vi "Configure Output Voltage.vi"(0 "VISA resource name":refnum<visa-resource-name>, 2 "Communication Address (0)":i16 max=254 format="%x", 7 "Output Voltage (0)":dbl min=0.0 max=18.0 format="%#.2g", 11 "error in (no error)":errorcluster) -> (4 "VISA resource name out":refnum<visa-resource-name>, 15 "error out":errorcluster)   [LabVIEW 2015, in "BK Precision 178XB Series.lvlib"]
doc: "This VI configures the output voltage. The valid range depends on the maximum output voltage set using <b>Configure Max Output Voltage.vi</b>."
uses:
  <instrlib>/BK Precision 178XB Series/BK Precision 178XB Series.lvlib
panel:
  # "(c) 2009 B&K PRECISION CORPORATION.  ALL RIGHTS RESERVED."
  # "Note:  The allowable Output Voltage to be set is based on the maximum output voltage configured using Configure Max Output Voltage.vi . Any values out of the maximum will not work."
  # "V"
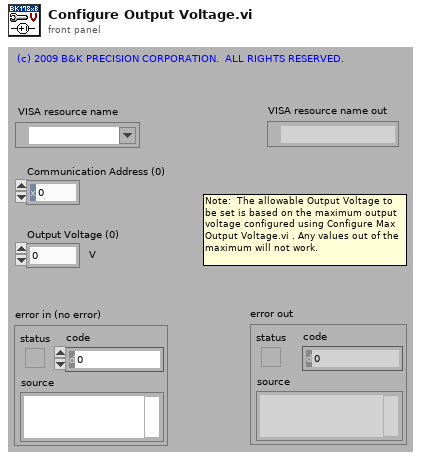
[diagram p1: front panel]
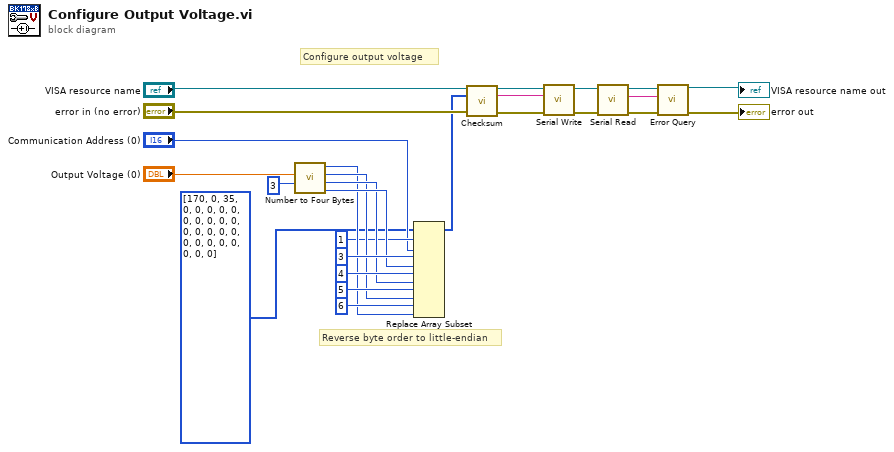
[diagram p0: block diagram]
diagram:
  # "Reverse byte order to little-endian"
  # "Configure output voltage"
  n1 = call <instrlib>:"Number to Four Bytes.vi"("Fractional Precision (3)"=3 ("index"), "Input Value (0)"="Output Voltage (0)") -> ("Byte 4"=w21:i32, "Byte 3"=w20:i32, "Byte 2"=w19:i32, "Byte 1"=w18:i32)  [unwired: 6 in]
  n2 = Replace Array Subset(array=i16[] [170, 0, 35, 0, 0, 0, 0, 0, 0, 0, 0, 0, 0, 0, 0, 0, 0, 0, 0, 0, 0, 0, 0, 0, 0, 0], new element #1="Communication Address (0)", index #1=1, new element #2=w21, index #2=3 ("index"), new element #3=w20, index #3=4 ("index"), new element #4=w19, index #4=5 ("index"), new element #5=w18, index #5=6 ("index")) -> (w1:i16[])
  n3 = call <instrlib>:"Checksum.vi"("VISA resource name"="VISA resource name", "Command Frame Array"=w1, "error in (no error)"="error in (no error)") -> ("VISA resource name out"=w8:refnum<visa-resource-name>, "Output String"=w6:string, "error out"=w7:errorcluster)  [unwired: 8 in, 2 out]
  n4 = call <instrlib>:"Serial Write.vi"("error in (no error)"=w7, "Input Command Frame"=w6, "VISA resource name"=w8) -> ("error out"=w17:errorcluster, "VISA resource name out"=w16:refnum<visa-resource-name>)  [unwired: 6 in, 1 out]
  n5 = call <instrlib>:"Serial Read.vi"("error in (no error)"=w17, "VISA resource name"=w16) -> ("error out"=w13:errorcluster, "Read Buffer"=w11:string, "VISA resource name out"=w12:refnum<visa-resource-name>)  [unwired: 7 in]
  n6 = call <instrlib>:"Error Query.vi"("VISA resource name"=w12, "Input Read Buffer 1"=w11, "error in (no error)"=w13) -> ("VISA resource name out"=→"VISA resource name out":refnum<visa-resource-name>, "error out"=→"error out":errorcluster)  [unwired: 7 in, 4 out]
